vi "NI9205_SUB-VI_SaveData.vi"(5 "Arraych6":dbl[](array[numeric]), 7 "Array Time":timestamp[](array[timestamp]), 8 "error in (no error)":errorcluster, 10 "Suffisso":string, 11 "file path (use dialog)":path) -> (0 "error out":errorcluster, 3 "LastSaved":string)   [LabVIEW 2020]
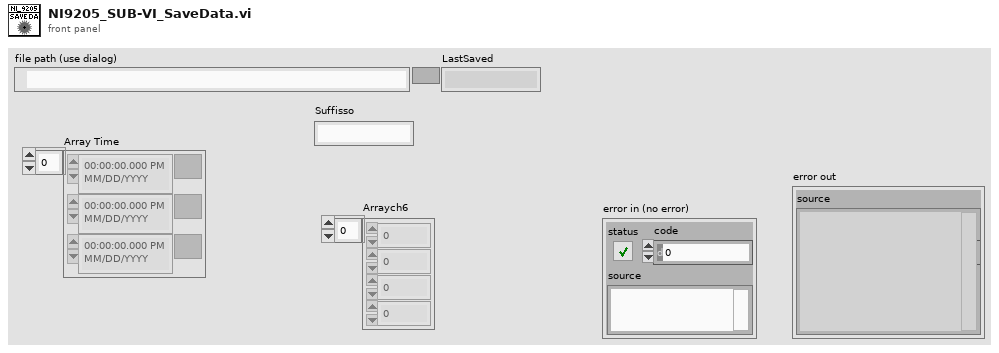
[diagram p1: front panel]
types:
  T1 = enum16{"open", "replace", "create", "open or create", "replace or create", "replace or create with confirmation"}
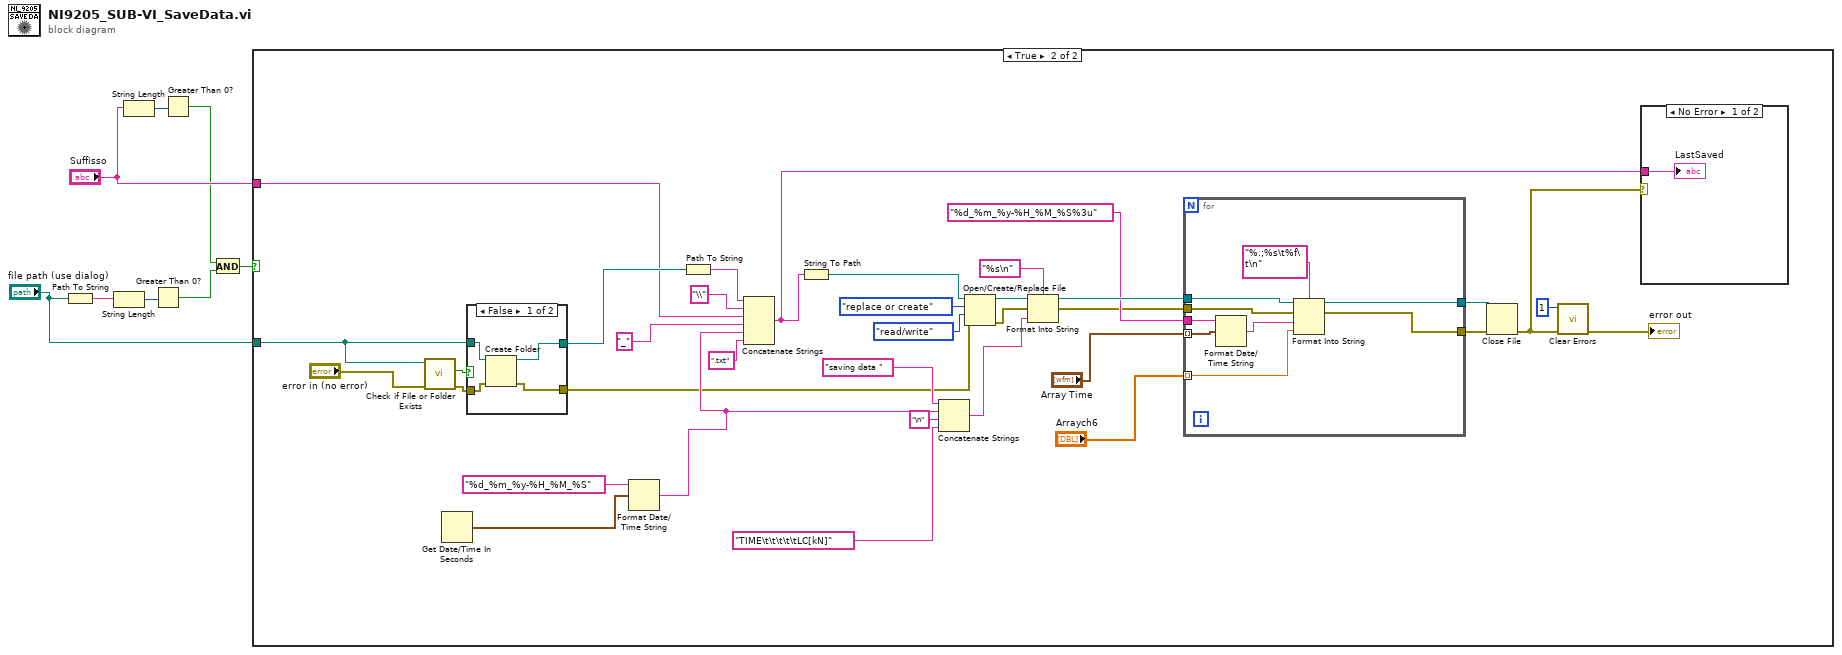
[diagram p0: block diagram]
diagram:
  n1 = Path To String(path="file path (use dialog)") -> (string=w4:string)
  n2 = String Length(string=w4) -> (length=w6:i32)
  n3 = String Length(string="Suffisso") -> (length=w7:i32)
  n4 = Greater Than 0?(x=w6) -> (x > 0?=w3:bool)
  n5 = Greater Than 0?(x=w7) -> (x > 0?=w2:bool)
  n6 = And(x=w2, y=w3) -> (x .and. y?=w1:bool)
  n7 = case shown="True" w1 {
    tunnel: "Suffisso" -> [_ w14]
    tunnel: "file path (use dialog)" -> [_ w9]
    frame False {
    }
    frame True {
      n8 = call <vilib>:"Check if File or Folder Exists.vi"("error in (no error)"="error in (no error)", "path"=w9) -> ("error out"=w16:errorcluster, "file or folder exists?"=w18:bool)  [unwired: 7 in, 1 out]
      n9 = Get Date/Time In Seconds() -> (seconds since 1Jan1904=w29:timestamp)
      n10 = case shown="False" w18 {
        tunnel: [w48 w50] -> w22
        tunnel: w16 -> [w45 w50]
        tunnel: w9 -> [w47 w49]
        tunnel: [w46 w49] -> w15
        frame False {
          n11 = Create Folder(path (use dialog)=w47, error in=w45) -> (created path=w46:path, error out=w48:errorcluster)  [unwired: 1 in, 1 out]
        }
        frame True {
        }
      }
      n12 = Format Date/Time String(time format string (%c)="%d_%m_%y-%H_%M_%S", seconds (now)=w29) -> (date/time string=w28:string)  [unwired: 1 in]
      n13 = Path To String(path=w15) -> (string=w33:string)
      n14 = Concatenate Strings(w33, "\\" ("string"), w14, "_" ("string"), w28, ".txt" ("string")) -> (w13:string)
      n15 = String To Path(string=w13) -> (path=w27:path)
      n16 = Concatenate Strings("saving data ", w28, "\n" ("string"), "TIME\t\t\t\t\tLC[kN]" ("string")) -> (w36:string)
      n17 = Open/Create/Replace File(file path (use dialog)=w27, error in=w22, operation (0:open)=T1."replace or create", access (0:read/write)=enum16{"read/write", "read-only", "write-only"}."read/write") -> (refnum out=w39:refnum<file>, error out=w21:errorcluster)  [unwired: 2 in, 1 out]
      n18 = Format Into String(format string="%s\n", initial string=w39, error in=w21, w36) -> (resulting string=w34:refnum<file>, error out=w20:errorcluster)
      n19 = for {
        tunnel: w34 -> [w59]
        tunnel: "Arraych6" -> [w53] mode=indexing
        tunnel: [w57] -> w40
        tunnel: "%d_%m_%y-%H_%M_%S%3u" ("time format string (%c)") -> [w56]
        tunnel: "Array Time" -> [w55] mode=indexing
        tunnel: w20 -> [w52]
        tunnel: [w51] -> w19
        n20 = Format Date/Time String(time format string (%c)=w56, seconds (now)=w55) -> (date/time string=w54:string)  [unwired: 1 in]
        n21 = Format Into String(format string="%.;%s\t%f\t\n", initial string=w59, error in=w52, w54, w53) -> (resulting string=w57:refnum<file>, error out=w51:errorcluster)
      }
      n22 = Close File(refnum=w40, error in=w19) -> (error out=w10:errorcluster)  [unwired: 1 out]
      n23 = call <vilib>:"Clear Errors.vi"("error in (no error)"=w10, "specific error code to clear (0: all)"=1) -> ("error out"=→"error out":errorcluster)  [unwired: 4 in, 1 out]
      n24 = case shown="No Error" w10 {
        tunnel: w13 -> [w44 _]
        frame No Error {
          "LastSaved" <- w44
        }
        frame Error {
        }
      }
    }
  }
